vi "user process.vi"(8 "error in":errorcluster, 11 "Parameters to process":T2) -> (0 "error out":errorcluster, 3 "Results from processing":T1)   [LabVIEW 2013, in "LED runtime.lvclass"]
uses:
  LED runtime.lvclass
  parameter user data.ctl
  result user data.ctl
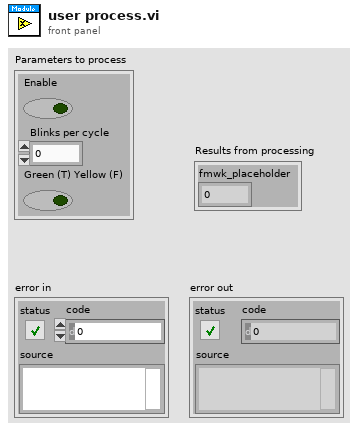
[diagram p1: front panel]
types:
  T1 = typedef "LED runtime.lvclass/result user data.ctl" = cluster{"fmwk_placeholder":i32}
  T2 = typedef "LED runtime.lvclass/parameter user data.ctl" = cluster{"Enable":bool, "Blinks per cycle":i32, "Green (T) Yellow (F)":bool}
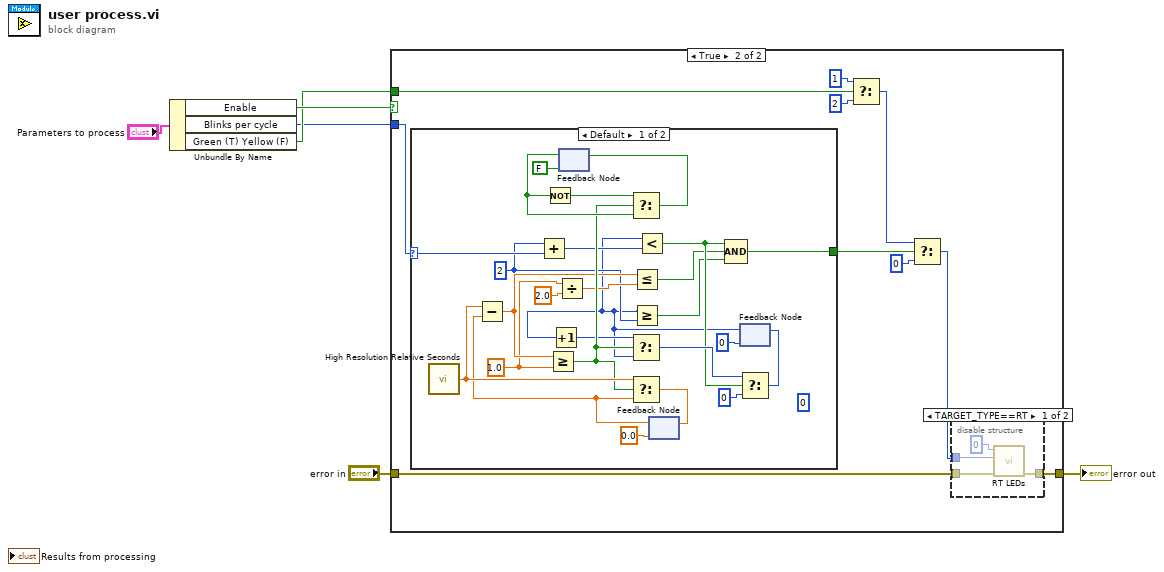
[diagram p0: block diagram]
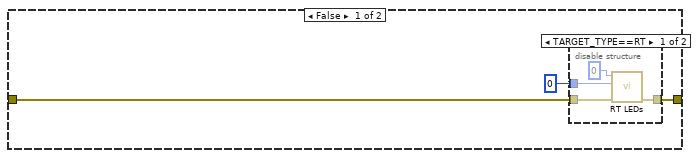
[diagram p2: hidden frame]
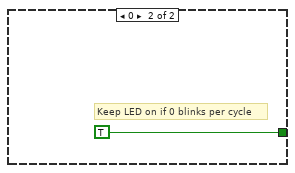
[diagram p4: hidden frame]
diagram:
  n1 = Unbundle By Name("Parameters to process") -> ("Enable"=w5:bool, "Blinks per cycle"=w1:i32, "Green (T) Yellow (F)"=w4:bool)
  n2 = case shown="True" w5 {
    tunnel: w4 -> [_ w23]
    tunnel: [w8 w17] -> w3
    tunnel: "error in" -> [w9 w16]
    tunnel: w1 -> [_ w14]
    frame False {
      n3 = disable-structure shown="TARGET_TYPE==RT" {
        disable-tunnel: 0 ("f") -> [w12 _]
        disable-tunnel: [w11 _] -> w8
        disable-tunnel: w9 -> [w10 _]
        frame condition #0 {
          n4 = call <vilib>:"RT LEDs.vi"("error in (no error)"=w10, "State"=w12, "LED Num"=0) -> ("error out"=w11:errorcluster)  [unwired: 3 in, 1 out]
        }
        frame condition #1 (active) {
        }
      }
    }
    frame True {
      n5 = case shown="Default" w14 {
        selector: w14 -> [w30 _]
        tunnel: [w33 TRUE] -> w15
        frame Default {
          w24 = 1.0
          (unwired) 0 ("f")
          w28 = 2 ("x")
          n6 = call <vilib>:"High Resolution Relative Seconds.vi"() -> ("relative seconds"=w44:dbl)
          n7 = Add(x=w28, y=w30) -> (x+y=w29:i32)
          n8 = Divide(x=w24, y=2.0) -> (x/y=w34:dbl)
          n9 = feedback #1(FALSE) -> (w45:bool)
          n10 = Not(x=w45) -> (.not. x?=w47:bool)
          n11 = feedback #2(0.0) -> (w43:dbl)
          n12 = Subtract(x=w44, y=w43) -> (x-y=w36:dbl)
          n13 = Greater Or Equal?(x=w36, y=w24) -> (x >= y?=w38:bool)
          n14 = Select(t=w47, s=w38, f=w45) -> (s? t:f=w46:bool)
          n15 = feedback-in #1(w46) -> ()
          n16 = Select(t=w44, s=w38, f=w43) -> (s? t:f=w42:dbl)
          n17 = Less Or Equal?(x=w36, y=w34) -> (x <= y?=w31:bool)
          n18 = feedback-in #2(w42) -> ()
          n19 = feedback #3(0 ("Blinks per cycle")) -> (w25:i32)
          n20 = Increment(x=w25) -> (x+1=w26:i32)
          n21 = Select(t=w26, s=w38, f=w25) -> (s? t:f=w37:i32)
          n22 = Greater Or Equal?(x=w25, y=w28) -> (x >= y?=w27:bool)
          n23 = Less?(x=w25, y=w29) -> (x < y?=w32:bool)
          n24 = Compound Arithmetic op=AND(w32, w31, w27) -> (w33:bool)
          n25 = Select(t=w37, s=w32, f=0) -> (s? t:f=w39:i32)
          n26 = feedback-in #3(w39) -> ()
        }
        frame 0 {
          # "Keep LED on if 0 blinks per cycle"
        }
      }
      n27 = Select(t=1 ("State"), s=w23, f=2 ("State")) -> (s? t:f=w20:i32)
      n28 = Select(t=w20, s=w15, f=0) -> (s? t:f=w18:i32)
      n29 = disable-structure shown="TARGET_TYPE==RT" {
        disable-tunnel: w18 -> [w53 _]
        disable-tunnel: [w52 _] -> w17
        disable-tunnel: w16 -> [w51 _]
        frame condition #0 {
          n30 = call <vilib>:"RT LEDs.vi"("error in (no error)"=w51, "State"=w53, "LED Num"=0) -> ("error out"=w52:errorcluster)  [unwired: 3 in, 1 out]
        }
        frame condition #1 (active) {
        }
      }
    }
  }
  "error out" <- w3
